vi "GUI Template.vi"(8 "Error In":errorcluster, 11 "Data In":T2) -> (0 "Error Out":errorcluster, 3 "Data Out":T2)   [LabVIEW 2019]
doc: "Description of VI"
uses:
  <vilib>/Utility/error.llb/DialogType.ctl
  <vilib>/Utility/miscctls.llb/LVPointTypeDef.ctl
  Controls/Data.ctl
panel:
  in  "Btn: Stop":bool
  out "Control Tab":T1(tab)
  out "Console Out":string
  out "Error Message":string
  out "VI-filename":string
  out "Revision Number":u32
  out "VI Description":string
  out "Callers' Names":string[](array[string])
  out "Code Size":u32
  out "VI Type":T3(ring)
  out "Project name":string
  out "Project filepath":path
  out "VI filepath":path
  out "Project Description":string
  out "VI-Name":string
  # "Common Errors:"
  # "0:"
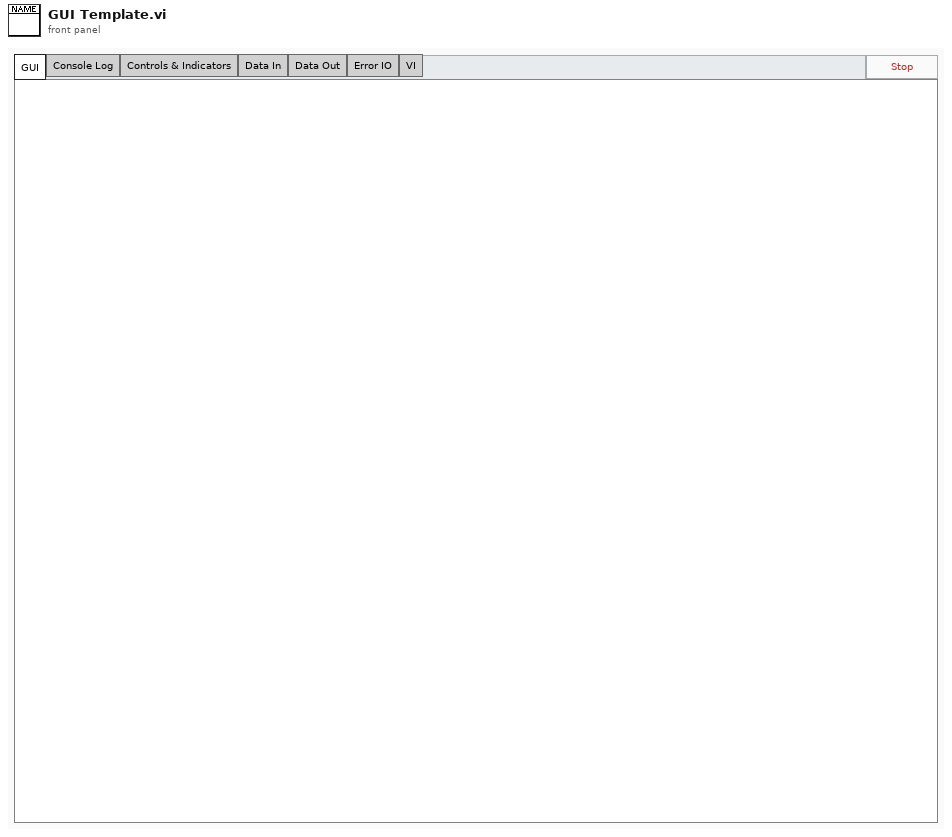
[diagram p1: front panel]
types:
  T1 = enum32{"GUI", "Console Log", "Controls & Indicators", "Data In", "Data Out", "Error IO", "VI"}
  T2 = typedef "Data.ctl" = cluster{"Log":string}
  T3 = enum32{"invalid VI type", "Standard VI", "Control VI", "Global VI", "Polymorphic VI", "Configuration VI", "SubSystem", "Facade VI", "Method VI", "Statechart Diagram VI"}
  T4 = enum32{"Invalid", "Standard", "Closed", "Hidden", "Minimized", "Maximized"}
  T5 = typedef "LVPointTypeDef.ctl" = cluster{"Horizontal":i16, "Vertical":i16}
  T6 = typedef "DialogType.ctl" = u16
  T7 = typedef "LVRectTypeDef.ctl" = cluster{"Left":i16, "Top":i16, "Right":i16, "Bottom":i16}
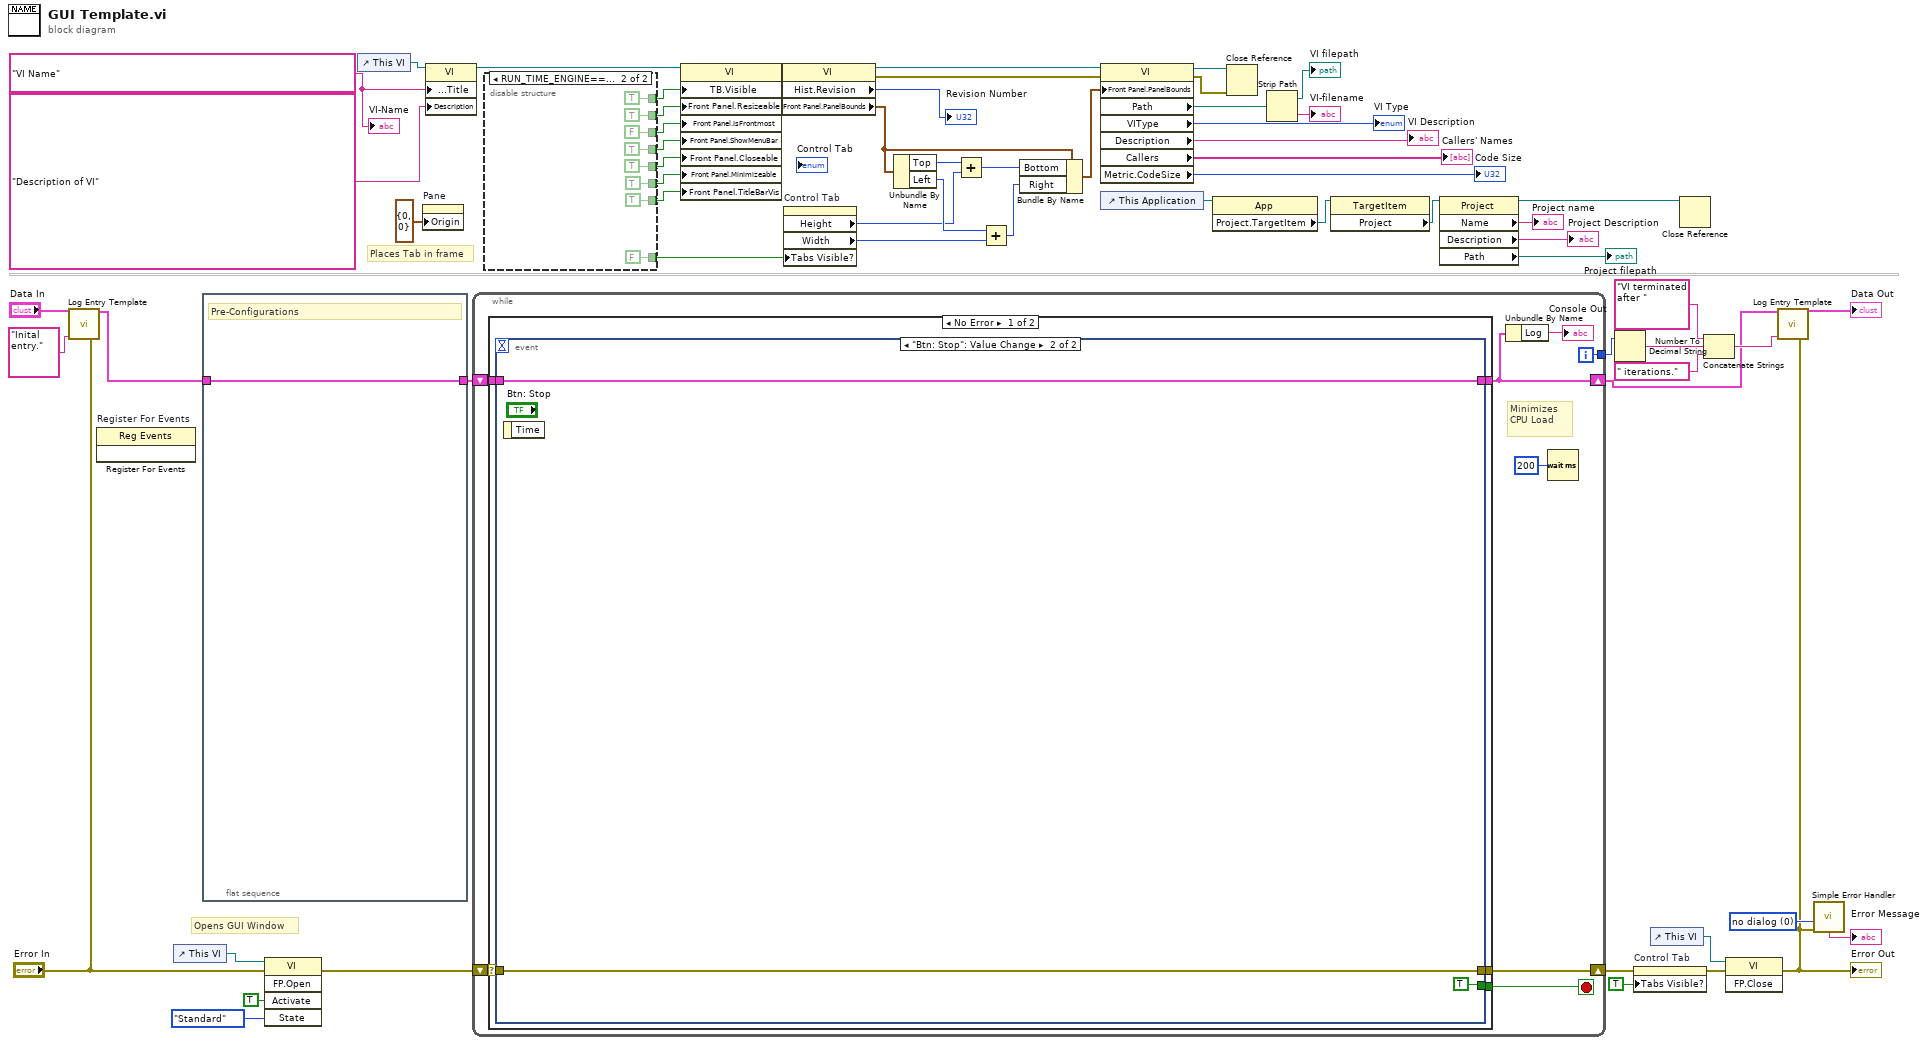
[diagram p0: block diagram]
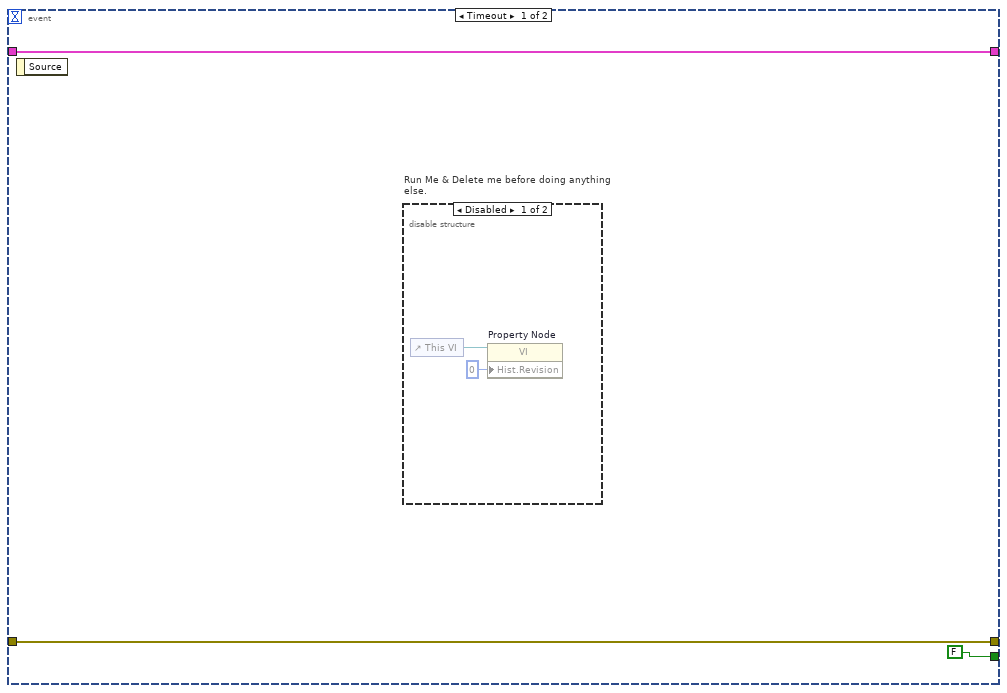
[diagram p2: hidden frame]
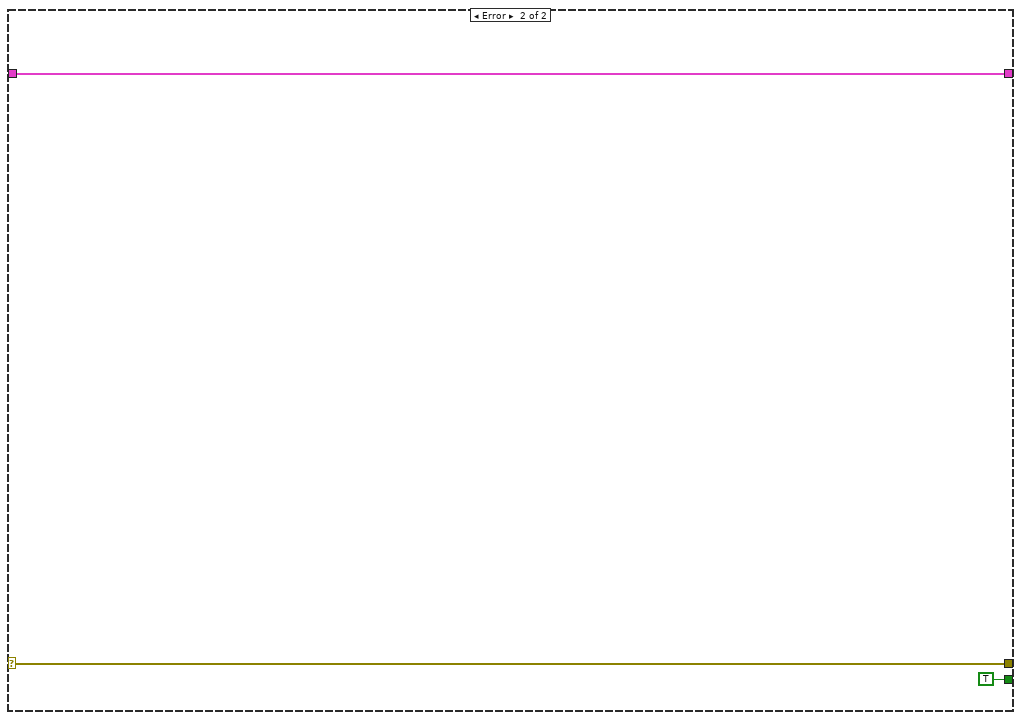
[diagram p4: hidden frame]
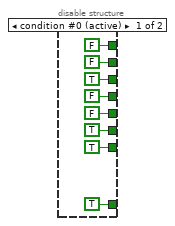
[diagram p5: hidden frame]
diagram:
  w34 = "VI Name"
  w62 = T6 0 items=["no dialog", "OK message", "continue or stop message", "OK message + warnings", "continue/stop + warnings"] ("type of dialog (OK msg:1)")
  # "Opens GUI Window"
  # "Places Tab in frame"
  n1 = call "Log Entry Template.vi"("Data In"="Data In", "Console Entry"="Inital entry.", "Error In"="Error In") -> ("Data Out"=w2:T2)  [unwired: 11 in, 1 out]
  n2 = register-events "Register For Events"() -> ()  [unwired: 3 in, 2 out]
  n3 = control-ref of="This VI"() -> (w12:refnum<vi>)
  n4 = flat-sequence {
    tunnel: w2 -> [w66]
    tunnel: [w66] -> w1
    frame #0 {
      # "Pre-Configurations"
    }
  }
  n5 = invoke on="Invoke Node" class="VI" method="FP.Open"(reference=w12, error in="Error In", "Activate"=TRUE ("Activate?"), "State"=T4."Standard") -> (error out=w9:errorcluster)  [unwired: 1 in, 4 out]
  n6 = control-ref of="This VI"() -> (w46:refnum<vi>)
  n7 = property on="Pane" class="Pane"("Origin"=T5 {"Horizontal"=0, "Vertical"=0}) -> ()  [unwired: 2 in, 2 out]
  n8 = property class="VI"(reference=w46, "Front Panel.Title"=w34, "Description"="Description of VI") -> (reference out=w36:refnum<vi>)  [unwired: 1 in, 1 out]
  n9 = while {
    shift-right: [w72] -> w7
    shift-left: w9 -> [w74]
    shift-right: [w69] -> w3
    shift-left: w1 -> [w71]
    tunnel: [w70] -> w17
    i -> [w70]
    stop <- w73 stop-if-true
    # "Minimizes CPU Load"
    n10 = case shown="No Error" w74 {
      selector: w74 -> [w78 w88]
      tunnel: [w77 TRUE] -> w73
      tunnel: [w79 w88] -> w72
      tunnel: w71 -> [w75 w89]
      tunnel: [w76 w89] -> w69
      frame No Error {
        n11 = event shown="[1] \"Btn: Stop\": Value Change" {
          selector: _ -> [_ _]
          dyn-events: _ -> [_ _]
          timeout: _ -> [_ _]
          tunnel: [w82 w85] -> w79
          tunnel: w78 -> [w82 w85]
          tunnel: [FALSE TRUE] -> w77
          tunnel: [w80 w87] -> w76
          tunnel: w75 -> [w80 w87]
          event Timeout {
            n12 = event-data() -> ()  [unwired: 1 in, 1 out]
            n13 = disable-structure "Run Me & Delete me before doing anything else." shown="Disabled" {
              frame Disabled {
                n14 = control-ref of="This VI"() -> (w84:refnum<vi>)
                n15 = property on="Property Node" class="VI"(reference=w84, "Hist.Revision"=u32 0 ("History:Revision Number")) -> ()  [unwired: 1 in, 2 out]
              }
              frame Enabled {
              }
            }
          }
          event "Btn: Stop": Value Change {
            n16 = event-data() -> ()  [unwired: 1 in, 1 out]
          }
        }
      }
      frame Error {
      }
    }
    n17 = Unbundle By Name(w69) -> ("Log"=→"Console Out":string)
    n18 = Wait (ms)(milliseconds to wait=u32 200) -> ()  [unwired: 1 out]
  }
  n19 = disable-structure "Exe vs Sim" shown="RUN_TIME_ENGINE==True" {
    disable-tunnel: [FALSE ("Tool Bar:Visible") TRUE ("Tool Bar:Visible")] -> w45
    disable-tunnel: [FALSE ("Front Panel Window:Resizable") TRUE ("Front Panel Window:Resizable")] -> w44
    disable-tunnel: [TRUE ("Front Panel Window:Is Frontmost") FALSE ("Front Panel Window:Is Frontmost")] -> w43
    disable-tunnel: [FALSE ("Front Panel Window:Show Menu Bar") TRUE ("Front Panel Window:Show Menu Bar")] -> w42
    disable-tunnel: [FALSE ("Front Panel Window:Closeable") TRUE ("Front Panel Window:Closeable")] -> w41
    disable-tunnel: [TRUE ("Front Panel Window:Title Bar Visible") TRUE ("Front Panel Window:Title Bar Visible")] -> w40
    disable-tunnel: [TRUE ("Front Panel Window:Minimizable") TRUE ("Front Panel Window:Minimizable")] -> w39
    disable-tunnel: [TRUE FALSE] -> w35
    frame condition #0 (active) {
    }
    frame condition #1 {
    }
  }
  n20 = property class="VI"(reference=w36, "TB.Visible"=w45, "Front Panel.Resizeable"=w44, "Front Panel.IsFrontmost"=w43, "Front Panel.ShowMenuBar"=w42, "Front Panel.Closeable"=w41, "Front Panel.Minimizeable"=w39, "Front Panel.TitleBarVis"=w40) -> (reference out=w38:refnum<vi>, error out=w37:errorcluster)  [unwired: 1 in]
  n21 = property class="VI"(reference=w38, error in=w37) -> (reference out=w52:refnum<vi>, error out=w48:errorcluster, "Hist.Revision"=→"Revision Number":u32, "Front Panel.PanelBounds"=w53:T7)
  n22 = property on="Control Tab" class="TabCtl (strict)"("Tabs Visible?"=w35) -> ("Height"=w55:u32, "Width"=w59:u32)  [unwired: 2 in, 2 out]
  n23 = Unbundle By Name(w53) -> ("Top"=w54:i16, "Left"=w58:i16)
  n24 = Add(x=w54, y=w55) -> (x+y=w56:u32)
  n25 = Add(x=w58, y=w59) -> (x+y=w57:u32)
  n26 = Bundle By Name(cluster=w53, "Bottom"=w56, "Right"=w57) -> (w51:T7)
  n27 = property on="Window size" class="VI"(reference=w52, error in=w48, "Front Panel.PanelBounds"=w51) -> (reference out=w60:refnum<vi>, error out=w49:errorcluster, "Path"=w33:path, "VIType"=→"VI Type":T3, "Description"=→"VI Description":string, "Callers"=→"Callers' Names":string[], "Metric.CodeSize"=→"Code Size":u32)
  n28 = control-ref of="This Application"() -> (w23:refnum<vi>)
  n29 = property class="App"(reference=w23) -> ("Project.TargetItem"=w28:refnum<vi>)  [unwired: 1 in, 2 out]
  n30 = Close Reference(reference=w60, error in (no error)=w49) -> ()  [unwired: 1 out]
  n31 = Strip Path(path=w33) -> (stripped path=→"VI filepath":path, name=→"VI-filename":string)
  n32 = property class="TargetItem"(reference=w28) -> ("Project"=w27:refnum<vi>)  [unwired: 1 in, 2 out]
  n33 = property class="Project"(reference=w27) -> (reference out=w21:refnum<vi>, "Name"=→"Project name":string, "Description"=→"Project Description":string, "Path"=→"Project filepath":path)  [unwired: 1 in, 1 out]
  n34 = Number To Decimal String(number=w17) -> (decimal integer string=w15:string)  [unwired: 1 in]
  n35 = property on="Control Tab" class="TabCtl (strict)"(error in=w7, "Tabs Visible?"=TRUE) -> (error out=w6:errorcluster)  [unwired: 1 in, 1 out]
  n36 = control-ref of="This VI"() -> (w4:refnum<vi>)
  n37 = Close Reference(reference=w21) -> ()  [unwired: 1 in, 1 out]
  n38 = Concatenate Strings("VI terminated after " ("Console Entry"), w15, " iterations.") -> (w13:string)
  n39 = invoke on="Invoke Node" class="VI" method="FP.Close"(reference=w4, error in=w6) -> (error out=w5:errorcluster)  [unwired: 1 in, 2 out]
  "Error Out" <- w5
  n40 = call "Log Entry Template.vi"("Data In"=w3, "Console Entry"=w13, "Error In"=w5) -> ("Data Out"=→"Data Out":T2)  [unwired: 11 in, 1 out]
  n41 = call <vilib>:"Simple Error Handler.vi"("type of dialog (OK msg:1)"=w62, "error in (no error)"=w5) -> ("message"=→"Error Message":string)  [unwired: 3 in, 4 out]
  "VI-Name" <- w34
